vi "GetPatternMatchResultNames.vi"(7 "ProjectName":string="Prj", 8 "error in (no error)":errorcluster, 10 "PatternMatchParameter":T1={"Algorithm"=2, "Match Parameters"={"Number of Matches Requested"=1, "Minimum Match Score"=750.0, "Angle Ranges"=[]}, "ROI Descriptor"={"Global Rectangle"=[], "Contours"=[]}, "Advanced Options"=[{"Item"=1, "Value"=1.0}, {"Item"=103, "Value"=1.0}], "Template path"="", "XOffset"=0, "YOffset"=0} {"ROI Descriptor"."Contours"."Type" items=["No Selection", "Point", "Line", "Rectangle", "Oval", "Polygon", "Freehand Region", "Annulus", "Unused2", "Unused3", "Broken Line", "Freehand Line", "Rotated Rectangle"]; "Advanced Options"."Item" items=["LD Sampling - Minimum Constrast"=0, "LD Sampling - Enable Subpixel Accuracy"=1, "LD Sampling - Search Strategy"=2, "LD Sampling - Subpixel Iterations"=3, "LD Sampling - Subpixel Tolerance"=4, "LD Sampling - Initial Match List Length"=5, "LD Sampling - Match List Reduction Factor"=6, "LD Sampling - Initial Step Size"=7, "LD Sampling - Intermediate Angular Accuracy"=8, "-"=9, "Pyramid - Max Pyramid Level"=100, "Pyramid - Minimum Contrast"=102, "Pyramid - Enable Subpixel Accuracy"=103, "Pyramid - Subpixel Iterations"=104, "Pyramid - Subpixel Tolerance"=105, "Pyramid - Initial Match List Length"=106, "Pyramid - Match List Reduction Factor"=107, "Pyramid - Intermediate Angular Accuracy"=108, "Pyramid - Process Border Matches"=109, "Pyramid - Min Match Separation Distance"=111, "Pyramid - Min Match Separation Angle"=112, "Pyramid - Max Match Overlap"=113, "Pyramid - Max Cache in MB"=114, "Pyramid - Clear Cache"=115]; "Match Parameters"."Angle Ranges"."End Angle" min=-360 max=360; "Match Parameters"."Angle Ranges"."Start Angle" min=-360 max=360; "Match Parameters"."Minimum Match Score" min=0 max=1000; "Match Parameters"."Number of Matches Requested" min=1 max=9999; "Algorithm" items=["All", "Low Discrepancy Sampling", "Grayscale Value Pyramid", "Gradients Pyramid"]}, 11 "ROI_Name":string="ROI1") -> (0 "error out":errorcluster, 3 "ResultNames":string[](array[string]))   [LabVIEW 2019]
uses:
  Controls/Parttern Match/Analysis_PatternMatch_Result.ctl
  Controls/Parttern Match/Analysis_PatternMatch_Parameter.ctl
panel:
  in  "Match":T3 {"Bounding Box"."y" format="%.2g"; "Bounding Box"."x" format="%.2g"; "Score" format="%.2f"; "Scale" format="%.2g"; "Angle" format="%.2g"; "Position"."y" format="%.2g"; "Position"."x" format="%.2g"}
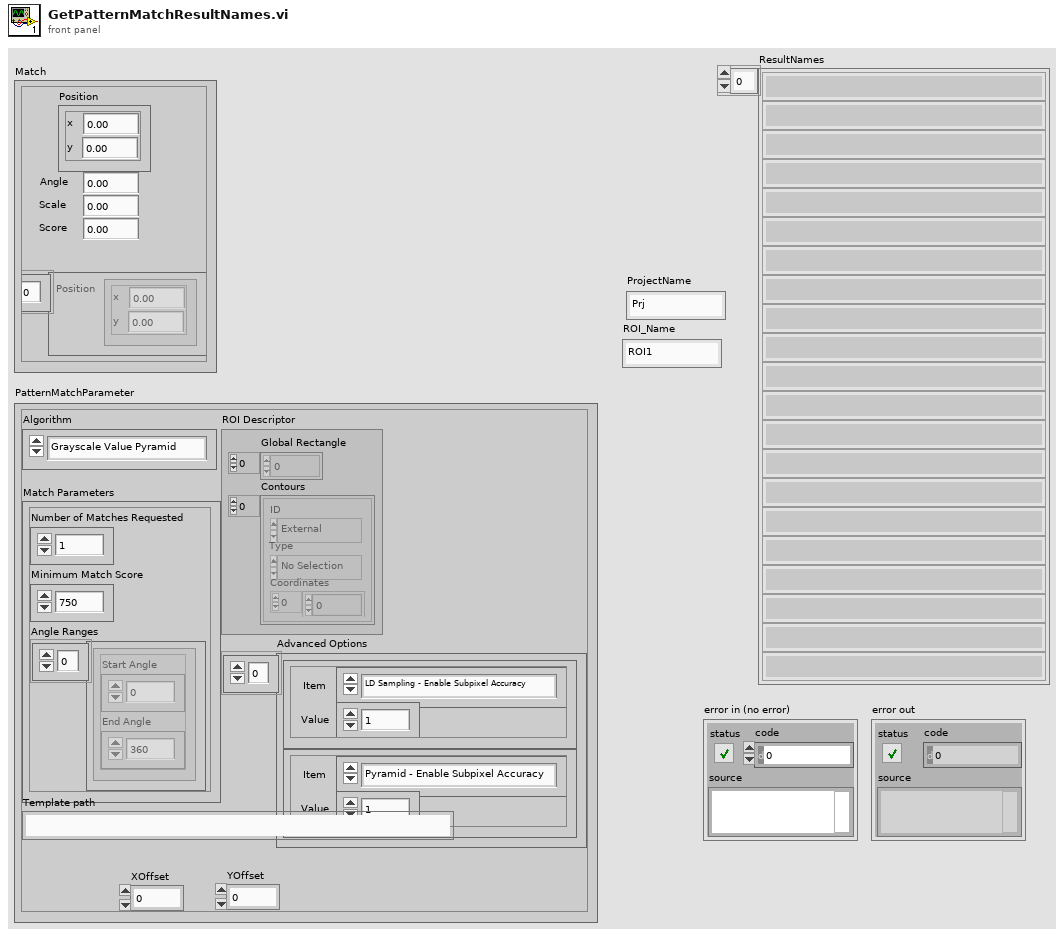
[diagram p1: front panel]
types:
  T1 = typedef "Analysis_PatternMatch_Parameter.ctl" = cluster{"Algorithm":i32, "Match Parameters":cluster{"Number of Matches Requested":i32, "Minimum Match Score":sgl, "Angle Ranges":cluster{"Start Angle":sgl, "End Angle":sgl}[]}, "ROI Descriptor":T2, "Advanced Options":cluster{"Item":u16, "Value":dbl}[], "Template path":string, "XOffset":i32, "YOffset":i32}
  T2 = typedef "ROI Descriptor" = cluster{"Global Rectangle":i32[], "Contours":cluster{"ID":enum32{"External", "Internal"}, "Type":u32, "Coordinates":i32[]}[]}
  T3 = typedef "Analysis_PatternMatch_Result.ctl" = cluster{"Position":cluster{"x":sgl, "y":sgl}, "Angle":sgl, "Scale":sgl, "Score":sgl, "Bounding Box":cluster{"x":sgl, "y":sgl}[]}
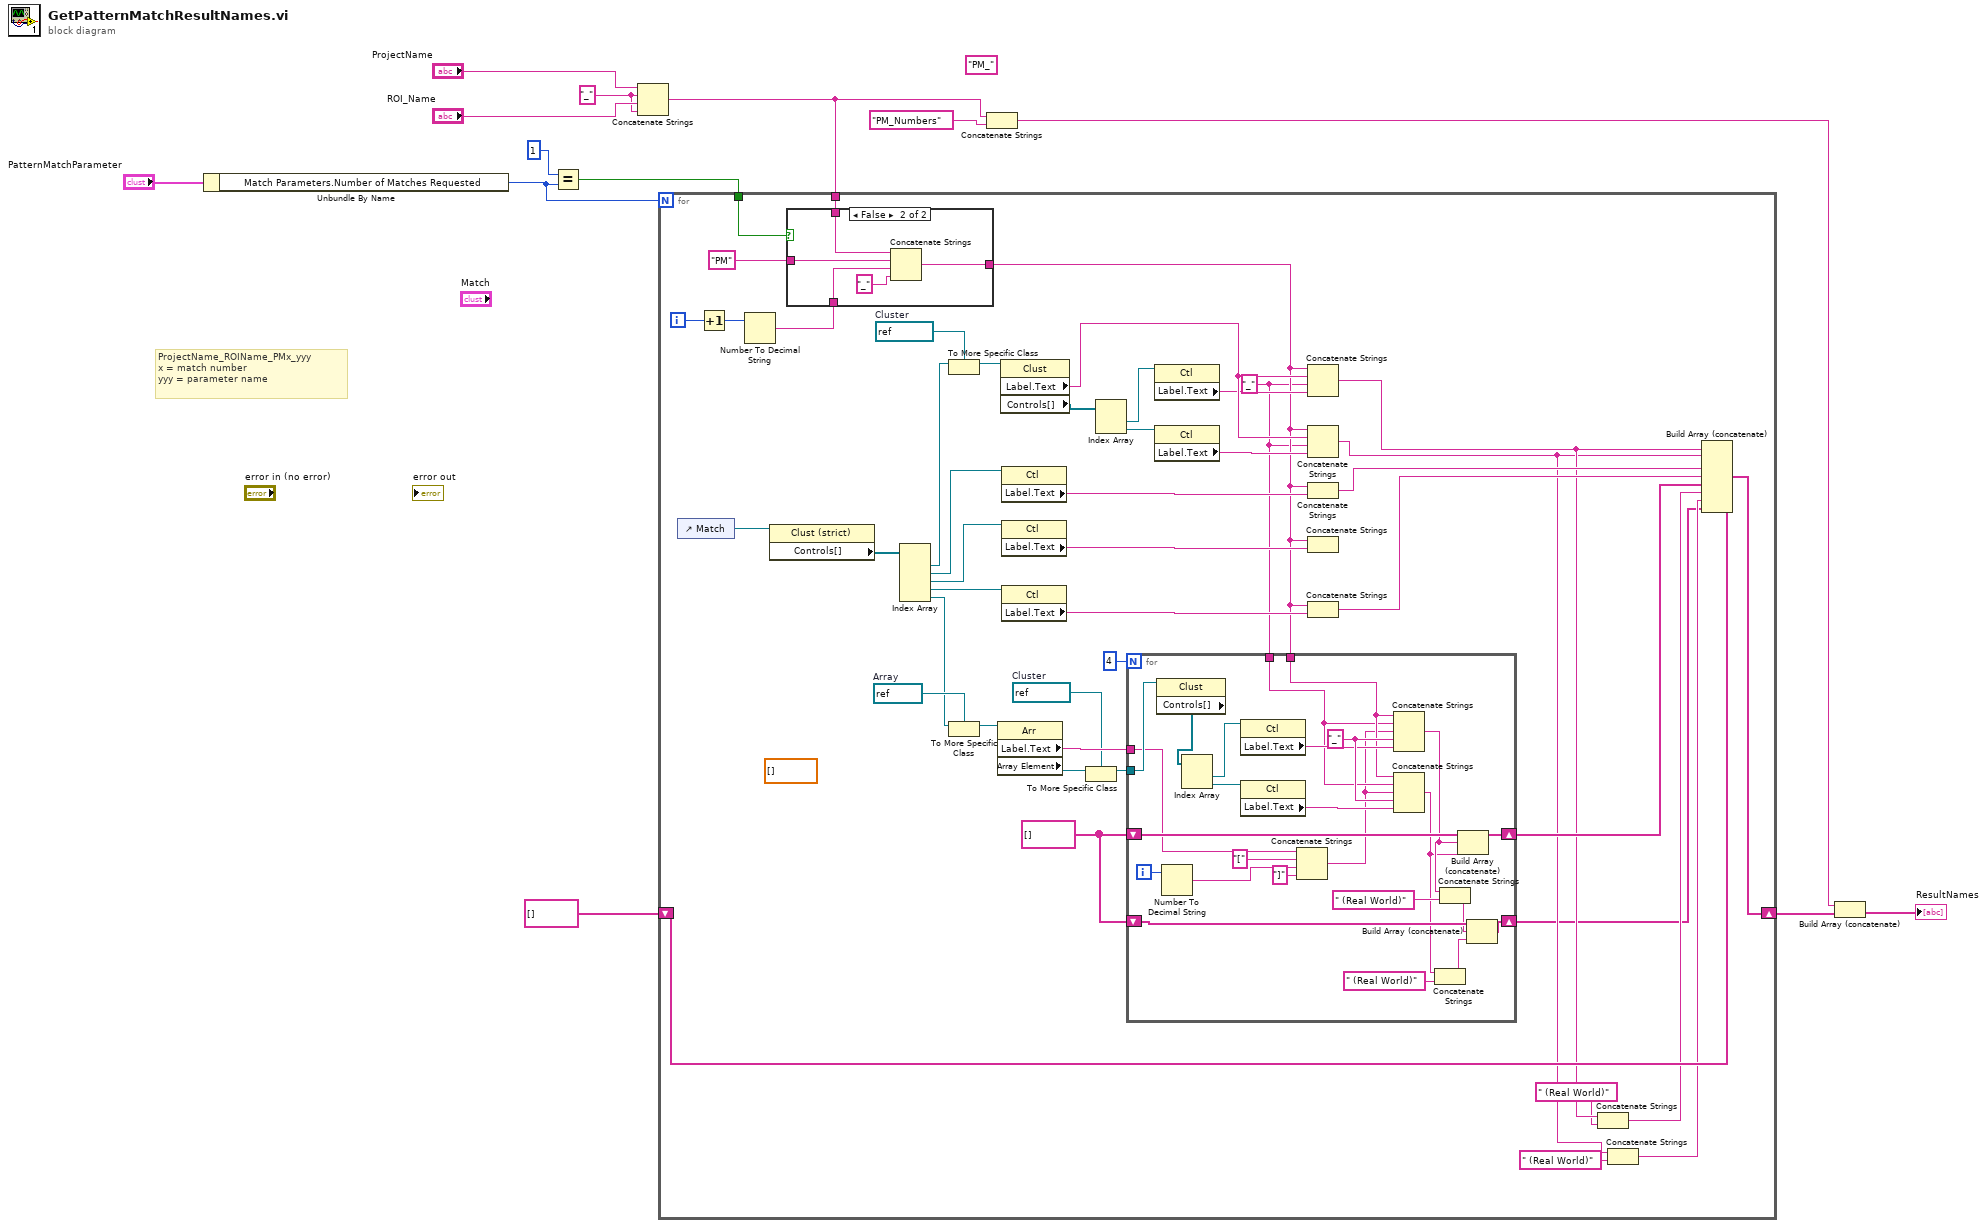
[diagram p0: block diagram]
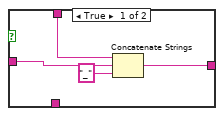
[diagram p2: hidden frame]
diagram:
  (unwired) "PM_" ("string")
  w9 = "_" ("string")
  # "ProjectName_ROIName_PMx_yyy\nx = match number\nyyy = parameter name"
  n1 = Unbundle By Name("PatternMatchParameter") -> ("Match Parameters.Number of Matches Requested"=w5:i32)
  n2 = Equal?(x=1, y=w5) -> (x = y?=w6:bool)
  n3 = Concatenate Strings("ProjectName", w9, "ROI_Name", w9) -> (w3:string)
  n4 = for {
    N: w5 -> [_]
    tunnel: w3 -> [w41]
    shift-right: [w43] -> w7
    shift-left: string[] [] -> [w44]
    tunnel: w6 -> [w42]
    i -> [w47]
    w17 = string[] []
    w27 = refnum<vi> refnum  # Cluster
    (unwired) dbl[] []
    w32 = refnum<vi> refnum  # Array
    w23 = "_" ("string")
    w55 = refnum<vi> refnum  # Cluster
    n5 = control-ref of="Match"() -> (w59:refnum<vi>)
    n6 = Increment(x=w47) -> (x+1=w46:i32)
    n7 = Number To Decimal String(number=w46) -> (decimal integer string=w40:string)  [unwired: 1 in]
    n8 = property class="Clust (strict)"(reference=w59) -> ("Controls[]"=w58:refnum<vi>[])  [unwired: 1 in, 2 out]
    n9 = case shown="False" w42 {
      tunnel: w41 -> [w88 w93]
      tunnel: w40 -> [_ w90]
      tunnel: [w87 w92] -> w24
      tunnel: "PM" ("string") -> [w86 w89]
      frame True {
        n10 = Concatenate Strings(w88, w86, "_" ("string")) -> (w87:string)
      }
      frame False {
        n11 = Concatenate Strings(w93, w89, w90, "_" ("string")) -> (w92:string)
      }
    }
    n12 = Index Array(array=w58) -> (element #1=w57:refnum<vi>, element #2=w38:refnum<vi>, element #3=w37:refnum<vi>, element #4=w48:refnum<vi>, element #5=w31:refnum<vi>)  [unwired: 5 in]
    n13 = To More Specific Class(target class=w55, reference=w57) -> (specific class reference=w56:refnum<vi>)  [unwired: 1 in, 1 out]
    n14 = To More Specific Class(target class=w32, reference=w31) -> (specific class reference=w30:refnum<vi>)  [unwired: 1 in, 1 out]
    n15 = property class="Arr"(reference=w30) -> ("Label.Text"=w29:string, "Array Element"=w26:refnum<vi>)  [unwired: 1 in, 2 out]
    n16 = property class="Clust"(reference=w56) -> ("Label.Text"=w51:string, "Controls[]"=w54:refnum<vi>[])  [unwired: 1 in, 2 out]
    n17 = property class="Ctl"(reference=w38) -> ("Label.Text"=w36:string)  [unwired: 1 in, 2 out]
    n18 = property class="Ctl"(reference=w37) -> ("Label.Text"=w35:string)  [unwired: 1 in, 2 out]
    n19 = property class="Ctl"(reference=w48) -> ("Label.Text"=w45:string)  [unwired: 1 in, 2 out]
    n20 = To More Specific Class(target class=w27, reference=w26) -> (specific class reference=w25:refnum<vi>)  [unwired: 1 in, 1 out]
    n21 = Index Array(array=w54) -> (element #1=w53:refnum<vi>, element #2=w52:refnum<vi>)  [unwired: 2 in]
    n22 = for {
      N: 4 -> [_]
      tunnel: w29 -> [w72]
      tunnel: w25 -> [w84]
      tunnel: w24 -> [w77]
      tunnel: w23 -> [w76]
      shift-right: [w74] -> w22
      shift-left: w17 -> [w75]
      shift-right: [w60] -> w14
      shift-left: w17 -> [w67]
      i -> [w73]
      w83 = "_" ("string")
      n23 = property class="Clust"(reference=w84) -> ("Controls[]"=w78:refnum<vi>[])  [unwired: 1 in, 2 out]
      n24 = Number To Decimal String(number=w73) -> (decimal integer string=w70:string)  [unwired: 1 in]
      n25 = Index Array(array=w78) -> (element #1=w79:refnum<vi>, element #2=w80:refnum<vi>)  [unwired: 2 in]
      n26 = property class="Ctl"(reference=w79) -> ("Label.Text"=w81:string)  [unwired: 1 in, 2 out]
      n27 = property class="Ctl"(reference=w80) -> ("Label.Text"=w82:string)  [unwired: 1 in, 2 out]
      n28 = Concatenate Strings(w72, "[" ("string"), w70, "]" ("string")) -> (w68:string)
      n29 = Concatenate Strings(w77, w76, w68, w83, w81) -> (w64:string)
      n30 = Concatenate Strings(w77, w76, w68, w83, w82) -> (w63:string)
      n31 = Concatenate Strings(w63, " (Real World)" ("string")) -> (w62:string)
      n32 = Concatenate Strings(w64, " (Real World)" ("string")) -> (w65:string)
      n33 = Build Array (concatenate)(w75, w64, w63) -> (w74:string[])
      n34 = Build Array (concatenate)(w67, w65, w62) -> (w60:string[])
    }
    n35 = property class="Ctl"(reference=w53) -> ("Label.Text"=w50:string)  [unwired: 1 in, 2 out]
    n36 = property class="Ctl"(reference=w52) -> ("Label.Text"=w49:string)  [unwired: 1 in, 2 out]
    n37 = Concatenate Strings(w24, w51, w23, w50) -> (w21:string)
    n38 = Concatenate Strings(w24, w51, w23, w49) -> (w18:string)
    n39 = Concatenate Strings(w24, w36) -> (w33:string)
    n40 = Concatenate Strings(w24, w35) -> ()  [unwired: 1 out]
    n41 = Concatenate Strings(w24, w45) -> (w34:string)
    n42 = Concatenate Strings(w21, " (Real World)" ("string")) -> (w16:string)
    n43 = Concatenate Strings(w18, " (Real World)" ("string")) -> (w15:string)
    n44 = Build Array (concatenate)(w44, w21, w18, w33, w34, w22, w16, w15, w14) -> (w43:string[])
  }
  n45 = Concatenate Strings(w3, "PM_Numbers" ("string")) -> (w1:string)
  n46 = Build Array (concatenate)(w1, w7) -> (→"ResultNames":string[])
